vi "Drive Controller.vi"(8 "error in":errorcluster) -> ()   [LabVIEW 2018]
doc: "This VI executes continuously carrying out the current operation and responding to updates or new operation requests. It will often contain the timing or control code that is difficult to place directly in TeleOp. This VI generally opens all sensors and motors and isolates the rest of the robot code from knowing implementation details of how the operations are carried out."
uses:
  <vilib>/Rock Robotics/WPI/Framework/Completion Status.ctl
  Drive Setpoints.ctl
  Drive Operations.ctl
  <vilib>/Rock Robotics/WPI/ThirdParty/Phoenix-LabVIEW/Motor Controller/Controls/CTRE_Phoenix_MotorControl_NeutralMode.ctl
  <vilib>/Rock Robotics/WPI/RobotDrive/WPI_RobotDriveOpen4MotorWithExistingMotors.vi
  Framework/Robot Global Data.vi
  <vilib>/addons/control/pid/pid.llb/PID (DBL).vi
  <vilib>/addons/control/pid/NI_PID_pid.lvlib
panel:
  in  "PID gains":T1={"proportional gain (Kc)"=0.009, "integral time (Ti, min)"=0.0, "derivative time (Td, min)"=0.0}
  in  "Interactive Values":T2
  in  "Buttons":cluster{"Execute Cmd":bool, "Abort Cmd":bool}
  out "Command Timing":cluster{"Start Time (ms)":u32, "Iterations":i32}
  out "Status":T4
  out "Setpoints":T5(graph)
  out "Current\nCmd":string
  # "Tip: The graph shows the motor setpoints. It may also be helpful to observe inputs and sensor values.\nYou may also want to display tuning or debugging controls."
  # "Interactive Command: You may fill in the settings for a command\nand schedule it with the Execute button. You can observe and abort\nany command while fine tuning the code for the controller."
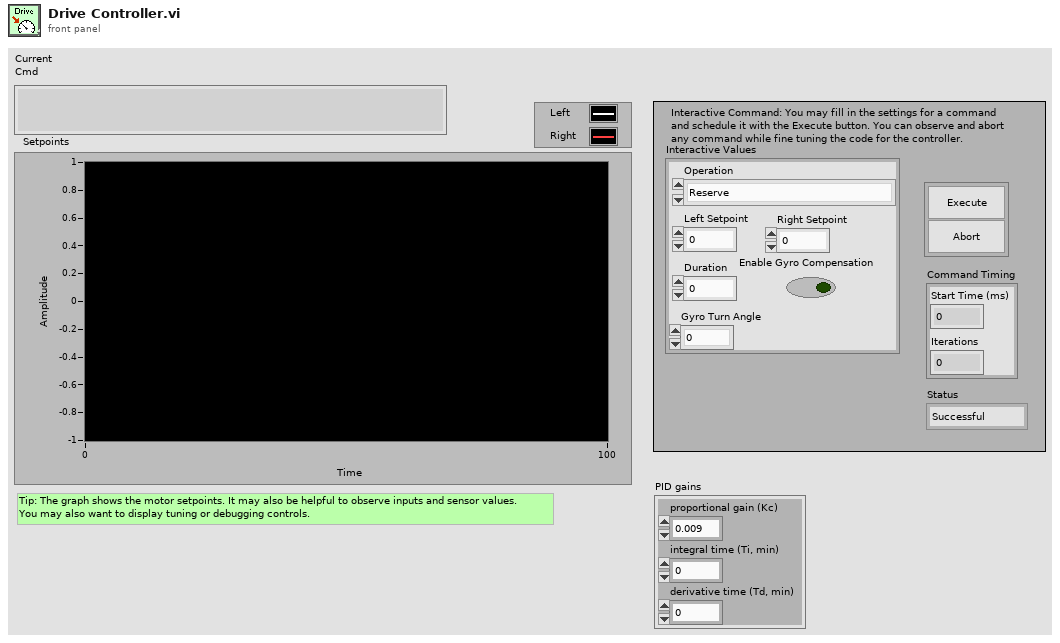
[diagram p1: front panel]
types:
  T1 = cluster{"proportional gain (Kc)":dbl, "integral time (Ti, min)":dbl, "derivative time (Td, min)":dbl}
  T2 = typedef "Drive Setpoints.ctl" = cluster{"Operation":T3, "Left Setpoint":dbl, "Right Setpoint":dbl, "Duration":dbl, "Enable Gyro Compensation":bool, "Gyro Turn Angle ":dbl}
  T3 = typedef "Drive Operations.ctl" = enum16{"Reserve", "Read Current", "Immediate", "Drive for Time", "Drive for Distance", "Gyro Turn"}
  T4 = typedef "Completion Status.ctl" = enum16{"Successful", "Aborted", "Incomplete"}
  T5 = cluster{"Left Setpoint":dbl, "Right Setpoint":dbl}
  T6 = typedef "CTRE_Phoenix_MotorControl_NeutralMode.ctl" = enum8{"EEPROMSetting", "Override to Coast", "Override to Brake"}
  T7 = typedef "WPI_MotorControlDeviceRef.ctl" = cluster{"DeviceStatus":errorcluster, "Type":T8, "PWM":cluster{"PWM Channel":T9, "DeadBand":T10}, "CAN":cluster{"Device Number":u8, "SetOutput VI Ref":variant, "GetOutput VI Ref":variant, "Enable VI Ref":variant, "Disable VI Ref":variant, "Data":variant}, "Invert":bool, "DIO PWM":cluster{"PWM \"Enable\" Channel":T9, "DIOChannel":T11, "PWM Rate":dbl}}
  T8 = typedef "WPI_MotorControlType.ctl" = enum16{"PWM", "CAN", "DIO PWM"}
  T9 = typedef "FPGA_DIOPWMChannel.ctl" = enum8{"PWM 0", "PWM 1", "PWM 2", "PWM 3", "PWM 4", "PWM 5", "PWM 6", "PWM 7", "PWM 8", "PWM 9", "PWM MXP 0", "PWM MXP 1", "PWM MXP 2", "PWM MXP 3", "PWM MXP 4", "PWM MXP 5", "PWM MXP 6", "PWM MXP 7", "PWM MXP 8", "PWM MXP 9", "Invalid"}
  T10 = typedef "WPI_PWMDeadband.ctl" = cluster{"Name":string, "maxPositivePwm":i32, "minPositivePwm":i32, "centerPwm":i32, "maxNegativePwm":i32, "minNegativePwm":i32, "angularRange":u16}
  T11 = typedef "FPGA_DIOChannel.ctl" = enum8{"DIO 0", "DIO 1", "DIO 2", "DIO 3", "DIO 4", "DIO 5", "DIO 6", "DIO 7", "DIO 8", "DIO 9", "DIO MXP 0", "DIO MXP 1", "DIO MXP 2", "DIO MXP 3", "DIO MXP 4", "DIO MXP 5", "DIO MXP 6", "DIO MXP 7", "DIO MXP 8", "DIO MXP 9", "DIO MXP 10", "DIO MXP 11", "DIO MXP 12", "DIO MXP 13", "DIO MXP 14", "DIO MXP 15", "SPI Port CS1", "SPI Port CS2", "SPI Port CS3", "SPI Port MISO", "SPI Port MOSI", "Invalid"}
  T12 = typedef "WPI_RobotDriveDevRef.ctl" = cluster{"DevStatus":errorcluster, "Motors[]":T7[], "Square Inputs":bool, "Max Output":dbl}
  T13 = typedef "Command Status Info.ctl" = cluster{"Name":string, "Status":T4, "notifier out":T14}
  T14 = typedef "Completion Notifier.ctl" = refnum<notifier>
  T15 = cluster{"SubSystem Data":T2, cluster{"Start Time (ms)":u32, "Iterations":i32}, cluster{"Command Info":T13, "Description":string, "Default Command":T2, "queue out":refnum<queue>, "Subsystem Name":string}}
  T16 = cluster{"X Angle":dbl, "Y Angle":dbl, "Z Angle":dbl}
  T17 = cluster{"SubSystem Data":T2, cluster{"Start Time (ms)":u32, "Iterations":i32}, "Default Command Arguments":cluster{"Command Info":T13, "Description":string, "Default Command":T2, "queue out":refnum<queue>, "Subsystem Name":string}}
  T18 = cluster{"LeftCompensatedSP":dbl, "RightCompensatedSP":dbl}
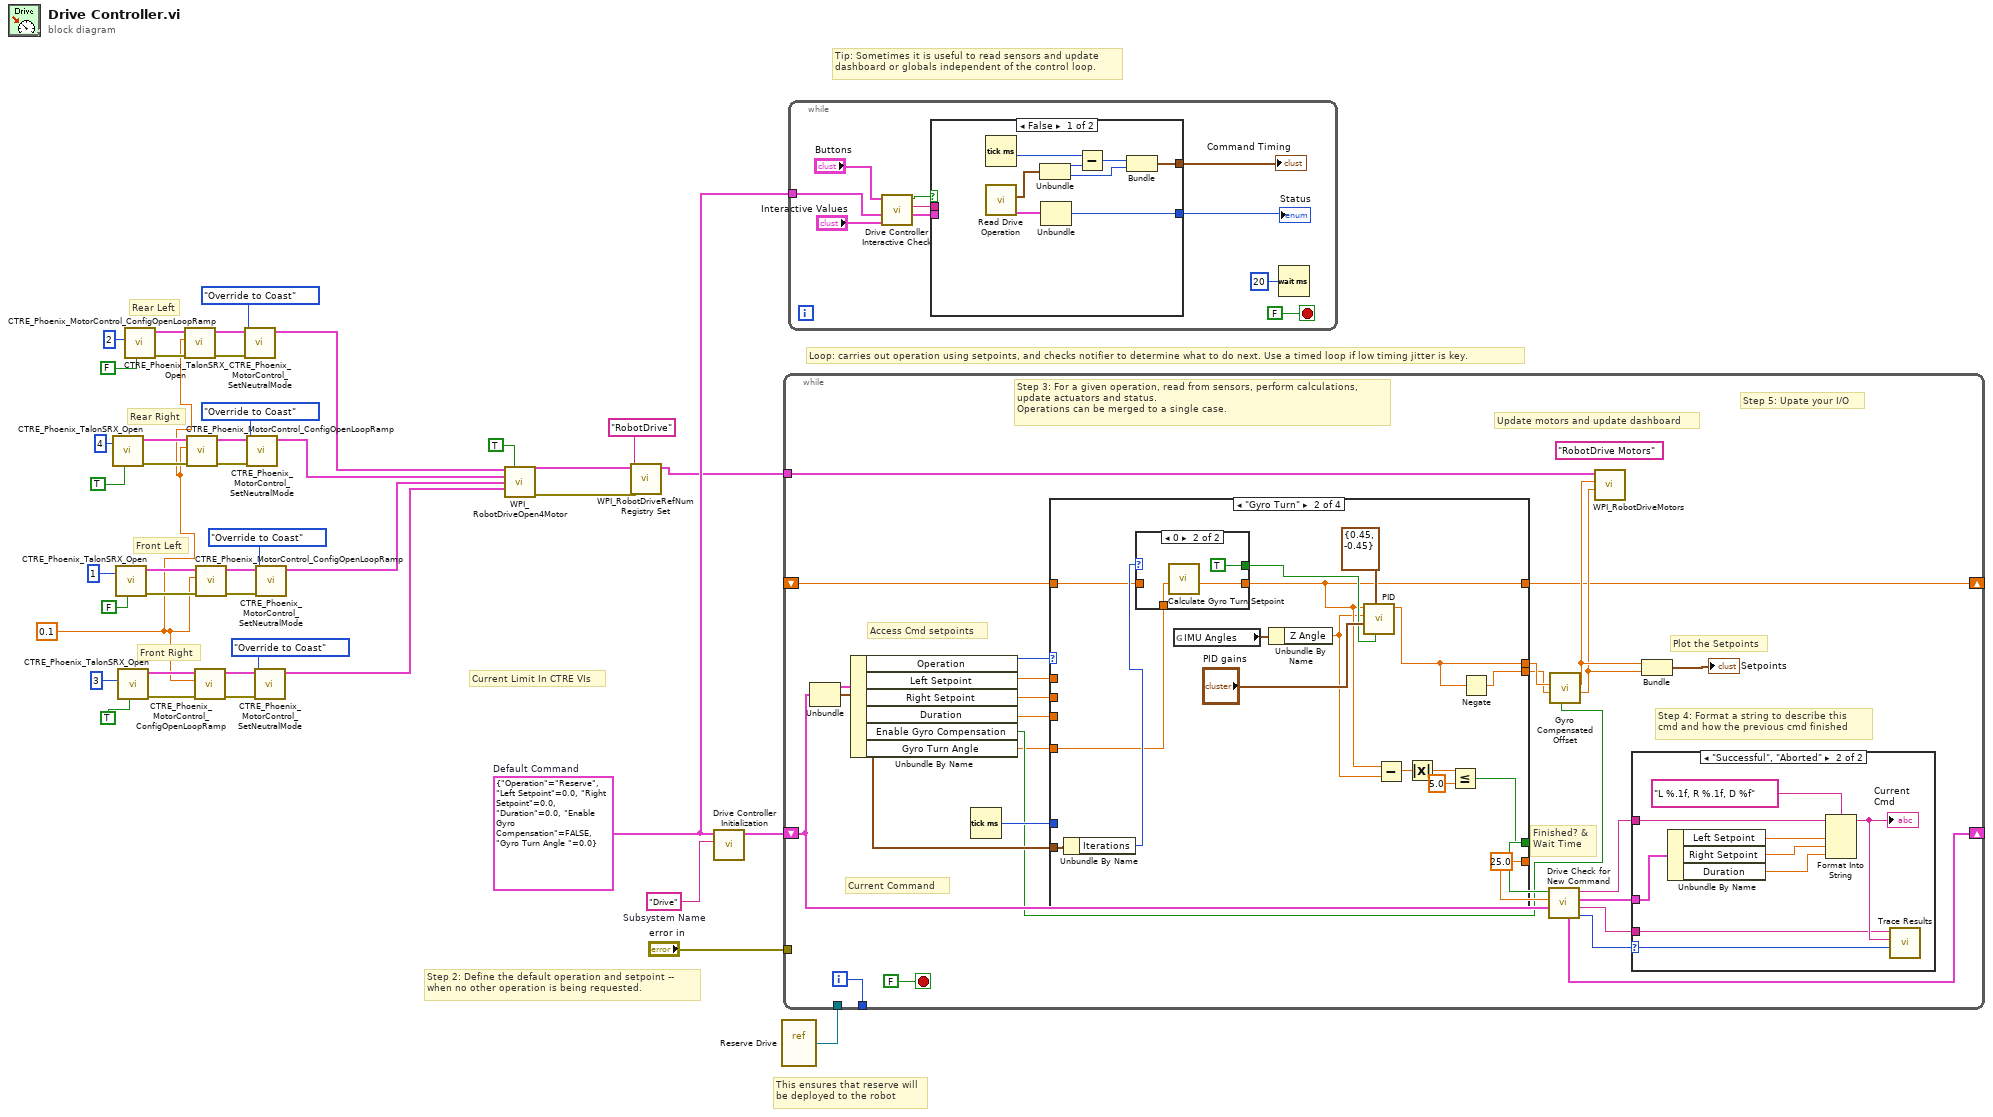
[diagram p0: block diagram]
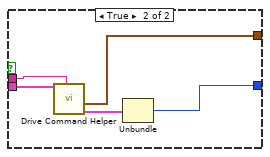
[diagram p2: hidden frame]
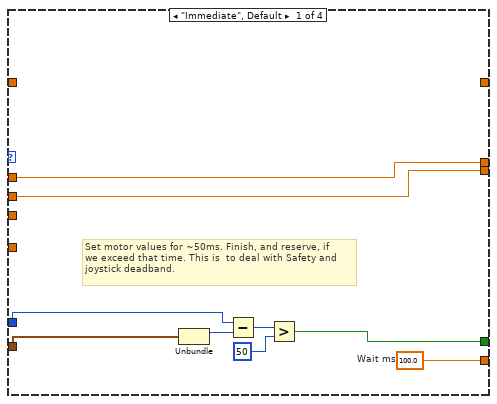
[diagram p4: hidden frame]
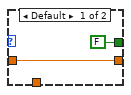
[diagram p5: hidden frame]
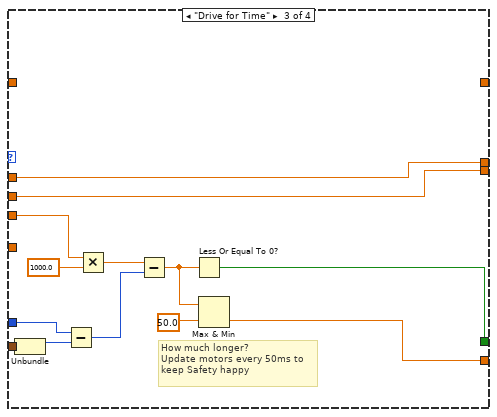
[diagram p6: hidden frame]
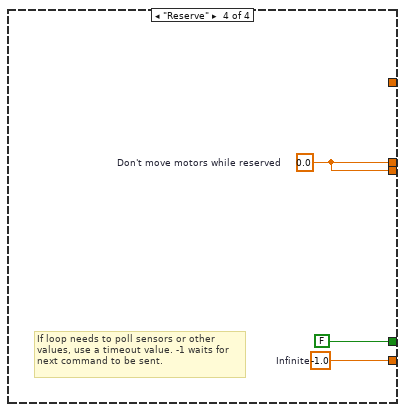
[diagram p7: hidden frame]
diagram:
  w3 = 0.1 ("secondsFromNeutralToFull")
  w39 = T2 {"Operation"=enum."Reserve", "Left Setpoint"=0.0, "Right Setpoint"=0.0, "Duration"=0.0, "Enable Gyro Compensation"=FALSE, "Gyro Turn Angle "=0.0}  # Default Command
  w43 = "Drive"  # Subsystem Name
  # "Rear Left"
  # "Rear Right"
  # "Front Left"
  # "Front Right"
  # "Current Limit In CTRE VIs"
  # "This ensures that reserve will\nbe deployed to the robot"
  # "Tip: Sometimes it is useful to read sensors and update\ndashboard or globals independent of the control loop."
  # "Step 2: Define the default operation and setpoint --\nwhen no other operation is being requested."
  # "Loop: carries out operation using setpoints, and checks notifier to determine what to do next. Use a timed loop if low timing jitter is key."
  n1 = call <vilib>:"CTRE_Phoenix_TalonSRX_Open.vi"("Invert"=TRUE, "Device Number"=u8 4) -> ("error out"=w19:errorcluster, "CAN Talon SRX Ref"=w24:T7)  [unwired: 8 in]
  n2 = call <vilib>:"CTRE_Phoenix_TalonSRX_Open.vi"("Invert"=FALSE, "Device Number"=u8 1) -> ("error out"=w20:errorcluster, "CAN Talon SRX Ref"=w26:T7)  [unwired: 8 in]
  n3 = call <vilib>:"CTRE_Phoenix_TalonSRX_Open.vi"("Invert"=TRUE, "Device Number"=u8 3) -> ("error out"=w30:errorcluster, "CAN Talon SRX Ref"=w31:T7)  [unwired: 8 in]
  n4 = call <vilib>:"CTRE_Phoenix_TalonSRX_Open.vi"("Invert"=FALSE, "Device Number"=u8 2) -> ("error out"=w14:errorcluster, "CAN Talon SRX Ref"=w16:T7)  [unwired: 8 in]
  n5 = call <vilib>:"CTRE_Phoenix_MotorControl_ConfigOpenLoopRamp.vi"("error in (no error)"=w14, "secondsFromNeutralToFull"=w3, "PhoenixMotorControlDevRef"=w16) -> ("error out"=w13:errorcluster, "PhoenixMotorControlDevRef"=w15:T7)  [unwired: 7 in]
  n6 = call <vilib>:"CTRE_Phoenix_MotorControl_ConfigOpenLoopRamp.vi"("error in (no error)"=w19, "secondsFromNeutralToFull"=w3, "PhoenixMotorControlDevRef"=w24) -> ("error out"=w18:errorcluster, "PhoenixMotorControlDevRef"=w23:T7)  [unwired: 7 in]
  n7 = call <vilib>:"CTRE_Phoenix_MotorControl_ConfigOpenLoopRamp.vi"("error in (no error)"=w30, "secondsFromNeutralToFull"=w3, "PhoenixMotorControlDevRef"=w31) -> ("error out"=w28:errorcluster, "PhoenixMotorControlDevRef"=w29:T7)  [unwired: 7 in]
  n8 = call <vilib>:"CTRE_Phoenix_MotorControl_ConfigOpenLoopRamp.vi"("error in (no error)"=w20, "secondsFromNeutralToFull"=w3, "PhoenixMotorControlDevRef"=w26) -> ("error out"=w21:errorcluster, "PhoenixMotorControlDevRef"=w25:T7)  [unwired: 7 in]
  n9 = call <vilib>:"CTRE_Phoenix_MotorControl_SetNeutralMode.vi"("error in (no error)"=w13, "Motor Control Neutral Mode"=CTRE_Phoenix_MotorControl_NeutralMode."Override to Coast", "PhoenixMotorControlDevRef"=w15) -> ("PhoenixMotorControlDevRef"=w33:T7)  [unwired: 7 in, 1 out]
  n10 = call <vilib>:"CTRE_Phoenix_MotorControl_SetNeutralMode.vi"("error in (no error)"=w18, "Motor Control Neutral Mode"=CTRE_Phoenix_MotorControl_NeutralMode."Override to Coast", "PhoenixMotorControlDevRef"=w23) -> ("PhoenixMotorControlDevRef"=w34:T7)  [unwired: 7 in, 1 out]
  n11 = call <vilib>:"CTRE_Phoenix_MotorControl_SetNeutralMode.vi"("error in (no error)"=w28, "Motor Control Neutral Mode"=CTRE_Phoenix_MotorControl_NeutralMode."Override to Coast", "PhoenixMotorControlDevRef"=w29) -> ("PhoenixMotorControlDevRef"=w36:T7)  [unwired: 7 in, 1 out]
  n12 = call <vilib>:"CTRE_Phoenix_MotorControl_SetNeutralMode.vi"("error in (no error)"=w21, "Motor Control Neutral Mode"=CTRE_Phoenix_MotorControl_NeutralMode."Override to Coast", "PhoenixMotorControlDevRef"=w25) -> ("PhoenixMotorControlDevRef"=w35:T7)  [unwired: 7 in, 1 out]
  n13 = call-poly <vilib>:"WPI_RobotDriveOpen4Motor.vi"("Rear Left Motor Dev Ref"=w33, "Square Inputs"=TRUE, "Rear Right Motor Dev Ref"=w34, "Front Left Motor Dev Ref"=w35, "Front Right Motor Dev Ref"=w36) -> ("RobotDriveDevRef"=w1:T12, "error out"=w32:errorcluster)  [unwired: 9 in]
  n14 = call <vilib>:"WPI_RobotDriveRefNum Registry Set.vi"("error in (no error)"=w32, "refnum name"="RobotDrive", "RobotDriveDevRef"=w1) -> ("RobotDriveDevRef"=w38:T12)  [unwired: 7 in, 1 out]
  n15 = call "Drive Controller Initialization.vi"("Subsystem Name"=w43, "Default Command"=w39) -> ("Current Command"=w41:T15)  [unwired: 9 in]
  n16 = vi-ref "Reserve Drive.vi"() -> (w40:refnum<vi>)
  n17 = while {
    shift-right: [w59] -> _
    shift-left: w41 -> [w52]
    tunnel: [w69] -> _
    tunnel: w38 -> [w67]
    tunnel: "error in" -> [_]
    tunnel: w40 -> [_]
    shift-right: [w45] -> _
    shift-left: _ -> [w44]
    i -> [w69]
    stop <- FALSE stop-if-true
    (unwired) "RobotDrive Motors" ("Name")
    # "Step 5: Upate your I/O"
    # "Step 4: Format a string to describe this\ncmd and how the previous cmd finished"
    # "Current Command"
    # "Update motors and update dashboard"
    # "Plot the Setpoints"
    # "Access Cmd setpoints"
    # "Finished? &\nWait Time"
    # "Step 3: For a given operation, read from sensors, perform calculations,\nupdate actuators and status.\nOperations can be merged to a single case."
    n18 = Unbundle(w52) -> ("SubSystem Data"=w66:T2, w53:cluster{"Start Time (ms)":u32, "Iterations":i32})  [unwired: 1 out]
    n19 = Unbundle By Name(w66) -> ("Operation"=w65:T3, "Left Setpoint"=w64:dbl, "Right Setpoint"=w63:dbl, "Duration"=w62:dbl, "Enable Gyro Compensation"=w51:bool, "Gyro Turn Angle"=w46:dbl)
    n20 = Tick Count (ms)() -> (millisecond timer value=w61:u32)
    n21 = case shown="\"Gyro Turn\"" w65 {
      tunnel: [w88 25.0 ("Infinite") w111 w126] -> w58
      tunnel: [w81 w93 w118 FALSE ("ignore previous (F)")] -> w57
      tunnel: w53 -> [w80 w105 w120 _]
      tunnel: [w87 w89 w117 w124] -> w50
      tunnel: [w86 w90 w116 w124] -> w49
      tunnel: w64 -> [w87 _ w117 _]
      tunnel: w63 -> [w86 _ w116 _]
      tunnel: w62 -> [_ _ w115 _]
      tunnel: w61 -> [w82 _ w114 _]
      tunnel: w46 -> [_ w103 _ _]
      tunnel: [_ w97 _ _] -> w45
      tunnel: w44 -> [_ w102 _ _]
      frame "Immediate", Default {
        w88 = 100.0  # Wait ms
        # "Set motor values for ~50ms. Finish, and reserve, if\nwe exceed that time. This is  to deal with Safety and\njoystick deadband."
        n22 = Unbundle(w80) -> ("Start Time (ms)"=w83:u32)  [unwired: 1 out]
        n23 = Subtract(x=w82, y=w83) -> (x-y=w84:u32)
        n24 = Greater?(x=w84, y=u8 50 ("Left Motor")) -> (0:w81:bool)
      }
      frame "Gyro Turn" {
        n25 = Unbundle By Name(w105) -> ("Iterations"=w104:i32)
        n26 = case shown="0" w104 {
          tunnel: w103 -> [_ w110]
          tunnel: [w107 w109] -> w97
          tunnel: w102 -> [w107 _]
          tunnel: [FALSE ("reinitialize? (F)") TRUE ("reinitialize? (F)")] -> w98
          frame Default {
          }
          frame 0 {
            n27 = call "Calculate Gyro Turn Setpoint.vi"("End Angle"=w110) -> ("Turn Setpoint"=w109:dbl)  [unwired: 10 in]
          }
        }
        n28 = global read "Robot Global Data.vi" "IMU Angles"() -> (w101:T16)
        n29 = Unbundle By Name(w101) -> ("Z Angle"=w96:dbl)
        n30 = call-poly <vilib>:"PID.vi"("reinitialize? (F)"=w98, "output range"=cluster{"output high":dbl, "output low":dbl} {"output high"=0.45, "output low"=-0.45}, "PID gains"="PID gains", "process variable"=w96, "setpoint"=w97) -> ("output"=w89:dbl)  [unwired: 5 in, 1 out]
        n31 = Subtract(x=w97, y=w96) -> (x-y=w95:dbl)
        n32 = Absolute Value(x=w95) -> (abs(x)=w94:dbl)
        n33 = Less Or Equal?(x=w94, y=5.0) -> (x <= y?=w93:bool)
        n34 = Negate(x=w89) -> (-x=w90:dbl)
      }
      frame "Drive for Time" {
        # "How much longer?\nUpdate motors every 50ms to\nkeep Safety happy"
        n35 = Unbundle(w120) -> ("Start Time (ms)"=w119:u32)  [unwired: 1 out]
        n36 = Subtract(x=w114, y=w119) -> (x-y=w123:u32)
        n37 = Multiply(x=w115, y=1000.0) -> (x*y=w122:dbl)
        n38 = Subtract(x=w122, y=w123) -> (x-y=w113:dbl)
        n39 = Less Or Equal To 0?(x=w113) -> (x <= 0?=w118:bool)
        n40 = Max & Min(x=w113, y=50.0) -> (min(x,y)=w111:dbl)  [unwired: 1 out]
      }
      frame "Reserve" {
        w124 = 0.0  # Don't move motors while reserved
        w126 = -1.0  # Infinite
        # "If loop needs to poll sensors or other\nvalues, use a timeout value. -1 waits for\nnext command to be sent."
      }
    }
    n41 = call "Drive Check for New Command.vi"("input cluster"=w52, "Wait time (ms)"=w58, "Finished?"=w57) -> ("Completion"=w60:T4, "Subsystem Name"=w54:string, "Current Command"=w55:T2, "Initial Trace String"=w56:string, "Next Command"=w59:T17)  [unwired: 4 in]
    n42 = call "Gyro Compensated Offset.vi"("Boolean"=w51, "Right Setpoint"=w49, "Left Setpoint"=w50) -> ("RightCompensatedSP"=w47:dbl, "LeftCompensatedSP"=w48:dbl)  [unwired: 7 in]
    n43 = call <vilib>:"WPI_RobotDriveMotors.vi"("RightSpeed"=w47, "LeftSpeed"=w48, "RobotDriveDevRef"=w67) -> ()  [unwired: 1 in, 8 out]
    n44 = case shown="\"Successful\", \"Aborted\"" w60 {
      selector: w60 -> [_ w79]
      tunnel: w56 -> [_ w74]
      tunnel: w55 -> [_ w75]
      tunnel: w54 -> [_ w71]
      frame "Incomplete", Default {
        # "Continuing current command"
      }
      frame "Successful", "Aborted" {
        # "Report and setup for next command"
        n45 = Unbundle By Name(w75) -> ("Left Setpoint"=w77:dbl, "Right Setpoint"=w78:dbl, "Duration"=w72:dbl)
        n46 = Format Into String(format string="L %.1f, R %.1f, D %f", initial string=w74, w77, w78, w72) -> (resulting string=w73:string)  [unwired: 1 in, 1 out]
        "Current\nCmd" <- w73
        n47 = call <vilib>:"Trace Results.vi"("Status of previous command"=w79, "Description"=w73, "Subsystem"=w71) -> ()  [unwired: 9 in]
      }
    }
    n48 = Bundle("LeftCompensatedSP"=w48, "RightCompensatedSP"=w47) -> (→"Setpoints":T18)  [unwired: 1 in]
  }
  n49 = while {
    tunnel: w39 -> [w128]
    stop <- FALSE stop-if-true
    n50 = call "Drive Controller Interactive Check.vi"("Interactive Command In"="Interactive Values", "Default Command"=w128, "Buttons"="Buttons") -> ("Interactive Command Out"=w130:T2, "Trace String"=w131:string, "Schedule"=w132:bool)  [unwired: 6 in]
    n51 = case shown="False" w132 {
      tunnel: [w141 w149] -> w133
      tunnel: [w140 w145] -> w134
      tunnel: w131 -> [_ w147]
      tunnel: w130 -> [_ w146]
      frame False {
        n52 = Tick Count (ms)() -> (millisecond timer value=w144:u32)
        n53 = call "Read Drive Operation.vi"() -> ("Command Info"=w138:T13, "Command Timing"=w137:cluster{"Start Time (ms)":u32, "Iterations":i32})  [unwired: 9 in, 1 out]
        n54 = Unbundle(w137) -> ("Start Time (ms)"=w142:u32, "Iterations"=w139:i32)
        n55 = Unbundle(w138) -> ("Status"=w141:T4)  [unwired: 2 out]
        n56 = Subtract(x=w144, y=w142) -> (x-y=w143:u32)
        n57 = Bundle(w143, "Iterations"=w139) -> (w140:cluster{u32, "Iterations":i32})  [unwired: 1 in]
      }
      frame True {
        n58 = call "Drive Command Helper.vi"("Description"=w147, "SubSystem Data"=w146) -> ("Command Info Out"=w148:T13, "Command Timing"=w145:cluster{"Start Time (ms)":u32, "Iterations":i32})  [unwired: 7 in, 1 out]
        n59 = Unbundle(w148) -> ("Status"=w149:T4)  [unwired: 2 out]
      }
    }
    "Status" <- w133
    "Command Timing" <- w134
    n60 = Wait (ms)(milliseconds to wait=u32 20) -> ()  [unwired: 1 out]
  }
